vi "LEBITplc.TestIonSourceSetValue.vi"(0 "i ref in":refnum<vi>, 1 "Nickname in":string, 2 "i attribute in":T1, 3 "index in":i32, 4 "value":dbl, 5 "error in":errorcluster) -> (13 "In Range?":bool, 14 "i ref out":refnum<vi>, 15 "Nicknames out":string[](array[string]), 16 "Index out":i32[](array[numeric]), 17 "values":dbl[](array[numeric]), 18 "Log Out":bool[](array[boolean]), 19 "error out":errorcluster)   [LabVIEW 2014, in "LEBITplc.lvlib"]
uses:
  LEBITplc.lvlib
  LEBITplc.i attribute.ctl
panel:
  in  "file path (dialog if empty)":path=path "\\\\Projects\\proj1/lebit/Data Exchange/data/IonGuideControl/Conversion/MassConversion.txt"
  out "i attribute out":T1
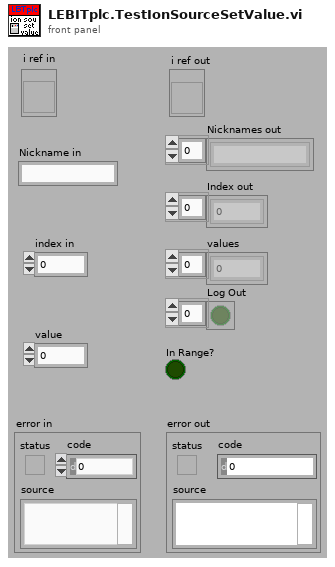
[diagram p1: front panel]
types:
  T1 = typedef "LEBITplc.lvlib/LEBITplc.i attribute.ctl" = cluster{"LLFLocation":string, "SetFileLocation":string, "nickNames":string[], "setValuePLCServiceID":i32[], "GUIServiceID":i32[], "monValuePLC":string[], "SetValueServiceID":i32[], "MonValueServiceID":i32[], "SetValue":dbl[][], "SetValueMin":dbl[], "SetValueMax":dbl[], "SetValueInfoServiceID":i32[], "GUINames":string[], "ListOfBases":string[], "Scale":dbl[], "Offset":dbl[], "setValuePLC":string[], "BaseName":string[], "ScaleServiceID":i32[], "OffsetServiceID":i32[], "AllPLCValues":string[], "CondSpecialArray":string[][], "CondSpecialIndex":i32[], "CondSpecialMonValue":dbl[], "RecentlyChanged":i32[], "SetFileLocationID":i32, "Dependent-Monitors":string[][], "LastLoadedFiles":string[], "IonGuideCalibLocation":string, "Monitor Dependent":string[], "Special":string[], "PLC?":bool[], "Start Date":string, "ListOfBasesServiceID":i32, "SETRA VISA resource":refnum<visa-resource-name>}
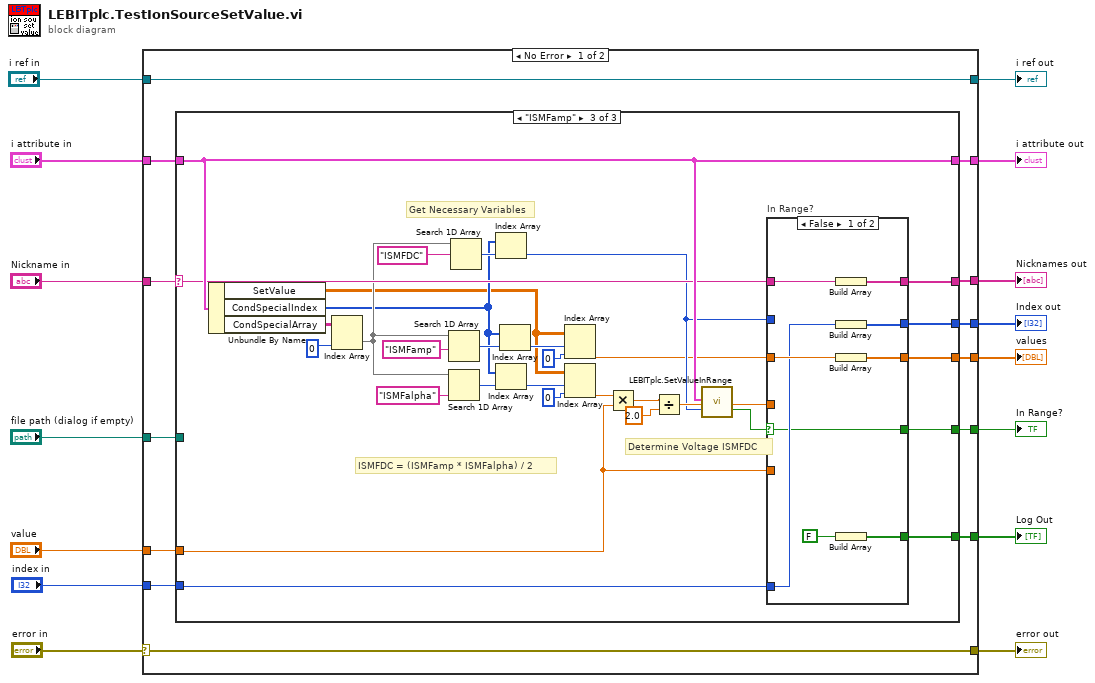
[diagram p0: block diagram]
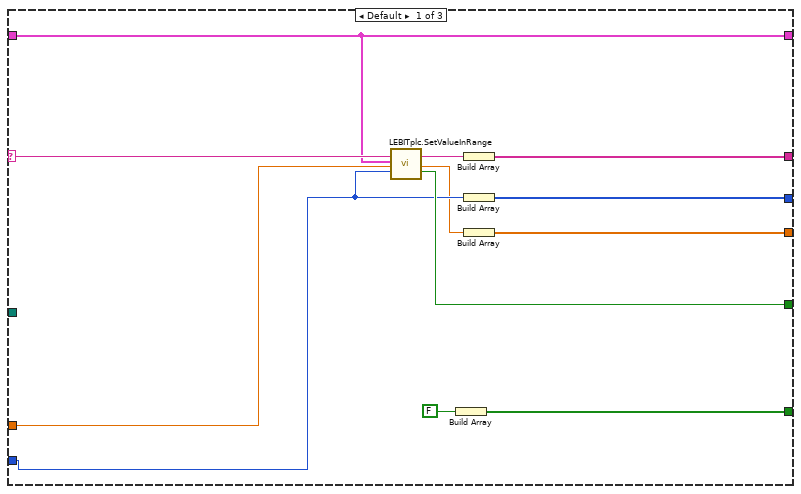
[diagram p2: hidden frame]
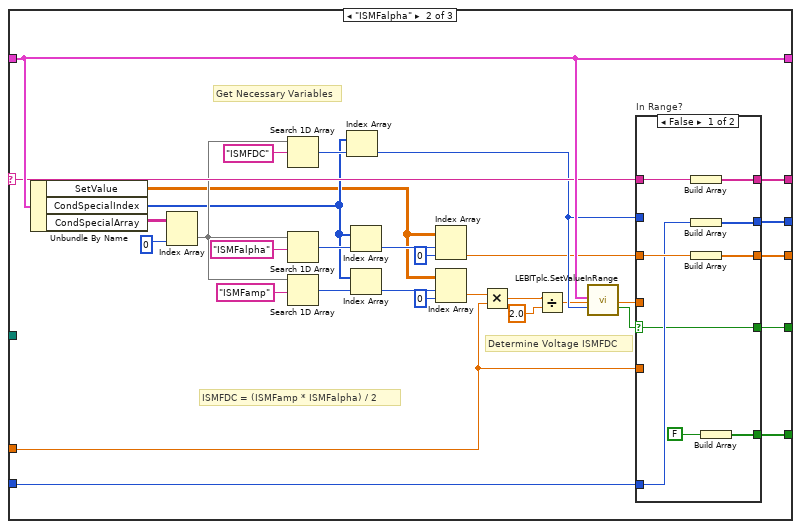
[diagram p3: hidden frame]
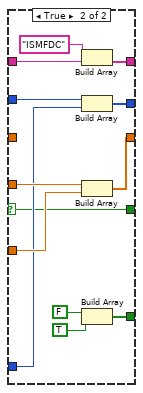
[diagram p4: hidden frame]
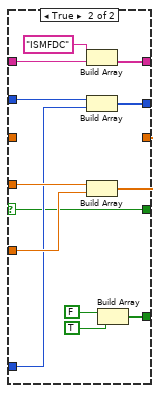
[diagram p5: hidden frame]
diagram:
  n1 = case shown="No Error" "error in" {
    selector: "error in" -> [w17 w151]
    tunnel: "Nickname in" -> [w28 _]
    tunnel: "i attribute in" -> [w27 w150]
    tunnel: "value" -> [w25 _]
    tunnel: [w24 _] -> w12
    tunnel: [w23 _] -> w3
    tunnel: "file path (dialog if empty)" -> [w22 _]
    tunnel: "index in" -> [w21 _]
    tunnel: [w20 _] -> w9
    tunnel: [w19 _] -> w8
    tunnel: [w18 _] -> w7
    tunnel: [w17 w151] -> w5
    tunnel: [w26 w150] -> w4
    tunnel: "i ref in" -> [w16 w149]
    tunnel: [w16 w149] -> w1
    frame No Error {
      n2 = case shown="\"ISMFamp\"" w28 {
        selector: w28 -> [w36 w67 w121]
        tunnel: w27 -> [w31 w72 w126]
        tunnel: [w31 w72 w126] -> w26
        tunnel: w25 -> [w34 w65 w105]
        tunnel: [w40 w68 w122] -> w24
        tunnel: [w39 w66 w120] -> w23
        tunnel: w22 -> [_ _ _]
        tunnel: w21 -> [w35 w57 w113]
        tunnel: [w38 w59 w114] -> w20
        tunnel: [w37 w55 w111] -> w19
        tunnel: [w29 w49 w103] -> w18
        frame Default {
          n3 = call "LEBITplc.SetValueInRange.vi"("CommandName in"=w36, "i attribute in"=w31, "value in"=w34, "index of element"=w35) -> ("CommandName out"=w32:string, "value out"=w33:dbl, "In Range?"=w37:bool)  [unwired: 11 in, 2 out]
          n4 = Build Array(FALSE) -> (w29:bool[])
          n5 = Build Array(w32) -> (w39:string[])
          n6 = Build Array(w35) -> (w38:i32[])
          n7 = Build Array(w33) -> (w40:dbl[])
        }
        frame "ISMFalpha" {
          # "ISMFDC = (ISMFamp * ISMFalpha) / 2"
          # "Determine Voltage ISMFDC"
          # "Get Necessary Variables"
          n8 = Unbundle By Name(w72) -> ("SetValue"=w42:dbl[][], "CondSpecialIndex"=w43:i32[], "CondSpecialArray"=w62:string[][])
          n9 = Index Array(array=w62, index (col)=0 ("index (row)")) -> (element=w44:string[])  [unwired: 1 in]
          n10 = Search 1D Array(1D array=w44, element="ISMFDC") -> (index of element=w63:i32)  [unwired: 1 in]
          n11 = Search 1D Array(1D array=w44, element="ISMFalpha") -> (index of element=w46:i32)  [unwired: 1 in]
          n12 = Search 1D Array(1D array=w44, element="ISMFamp") -> (index of element=w61:i32)  [unwired: 1 in]
          n13 = Index Array(array=w43, index=w63) -> (element=w58:i32)
          n14 = Index Array(array=w43, index=w46) -> (element=w45:i32)
          n15 = Index Array(array=w43, index=w61) -> (element=w60:i32)
          n16 = Index Array(array=w42, index (row)=w45, index (col)=0 ("disabled index (col)")) -> (element=w41:dbl)
          n17 = Index Array(array=w42, index (row)=w60, index (col)=0 ("disabled index (col)")) -> (element=w54:dbl)
          n18 = Multiply(x=w54, y=w65) -> (x*y=w52:dbl)
          n19 = Divide(x=w52, y=2.0) -> (x/y=w50:dbl)
          n20 = call "LEBITplc.SetValueInRange.vi"("i attribute in"=w72, "value in"=w50, "index of element"=w58) -> ("value out"=w69:dbl, "In Range?"=w53:bool)  [unwired: 12 in, 3 out]
          n21 = case "In Range?" shown="False" w53 {
            selector: w53 -> [w75 w85]
            tunnel: w41 -> [w81 _]
            tunnel: w65 -> [_ w93]
            tunnel: w69 -> [_ w94]
            tunnel: [w80 w92] -> w68
            tunnel: w67 -> [w78 w90]
            tunnel: [w79 w89] -> w66
            tunnel: [w77 w88] -> w59
            tunnel: w58 -> [_ w87]
            tunnel: w57 -> [w76 w86]
            tunnel: [w75 w85] -> w55
            tunnel: [w74 w82] -> w49
            frame False {
              n22 = Build Array(w78) -> (w79:string[])
              n23 = Build Array(w76) -> (w77:i32[])
              n24 = Build Array(w81) -> (w80:dbl[])
              n25 = Build Array(FALSE) -> (w74:bool[])
            }
            frame True {
              n26 = Build Array("ISMFDC" ("element"), w90) -> (w89:string[])
              n27 = Build Array(w87, w86) -> (w88:i32[])
              n28 = Build Array(w94, w93) -> (w92:dbl[])
              n29 = Build Array(FALSE ("element"), TRUE) -> (w82:bool[])
            }
          }
        }
        frame "ISMFamp" {
          # "ISMFDC = (ISMFamp * ISMFalpha) / 2"
          # "Get Necessary Variables"
          # "Determine Voltage ISMFDC"
          n30 = Unbundle By Name(w126) -> ("SetValue"=w96:dbl[][], "CondSpecialIndex"=w97:i32[], "CondSpecialArray"=w117:string[][])
          n31 = Index Array(array=w117, index (col)=0 ("index (row)")) -> (element=w98:string[])  [unwired: 1 in]
          n32 = Search 1D Array(1D array=w98, element="ISMFamp") -> (index of element=w100:i32)  [unwired: 1 in]
          n33 = Search 1D Array(1D array=w98, element="ISMFalpha") -> (index of element=w116:i32)  [unwired: 1 in]
          n34 = Search 1D Array(1D array=w98, element="ISMFDC") -> (index of element=w118:i32)  [unwired: 1 in]
          n35 = Index Array(array=w97, index=w118) -> (element=w104:i32)
          n36 = Index Array(array=w97, index=w116) -> (element=w115:i32)
          n37 = Index Array(array=w97, index=w100) -> (element=w99:i32)
          n38 = Index Array(array=w96, index (row)=w99, index (col)=0 ("disabled index (col)")) -> (element=w95:dbl)
          n39 = Index Array(array=w96, index (row)=w115, index (col)=0 ("disabled index (col)")) -> (element=w110:dbl)
          n40 = Multiply(x=w110, y=w105) -> (x*y=w108:dbl)
          n41 = Divide(x=w108, y=2.0) -> (x/y=w106:dbl)
          n42 = call "LEBITplc.SetValueInRange.vi"("i attribute in"=w126, "value in"=w106, "index of element"=w104) -> ("value out"=w123:dbl, "In Range?"=w109:bool)  [unwired: 12 in, 3 out]
          n43 = case "In Range?" shown="False" w109 {
            selector: w109 -> [w129 w139]
            tunnel: w95 -> [w135 _]
            tunnel: w105 -> [_ w147]
            tunnel: w123 -> [_ w148]
            tunnel: [w134 w146] -> w122
            tunnel: w121 -> [w132 w144]
            tunnel: [w133 w143] -> w120
            tunnel: [w131 w142] -> w114
            tunnel: w104 -> [_ w141]
            tunnel: w113 -> [w130 w140]
            tunnel: [w129 w139] -> w111
            tunnel: [w127 w136] -> w103
            frame False {
              n44 = Build Array(w132) -> (w133:string[])
              n45 = Build Array(w130) -> (w131:i32[])
              n46 = Build Array(w135) -> (w134:dbl[])
              n47 = Build Array(FALSE) -> (w127:bool[])
            }
            frame True {
              n48 = Build Array("ISMFDC" ("element"), w144) -> (w143:string[])
              n49 = Build Array(w141, w140) -> (w142:i32[])
              n50 = Build Array(w148, w147) -> (w146:dbl[])
              n51 = Build Array(FALSE, TRUE ("element")) -> (w136:bool[])
            }
          }
        }
      }
    }
    frame Error {
    }
  }
  "i attribute out" <- w4
  "values" <- w12
  "Nicknames out" <- w3
  "Index out" <- w9
  "In Range?" <- w8
  "Log Out" <- w7
  "error out" <- w5
  "i ref out" <- w1
